vi "2.vi"() -> ()   [LabVIEW 2018]
uses:
  <vilib>/DAQmx/read.llb/DAQmx Read (Analog DBL 1Chan 1Samp).vi
  <vilib>/DAQmx/write.llb/DAQmx Write (Digital Bool 1Line 1Point).vi
  <vilib>/DAQmx/create/channels.llb/DAQmx Create Channel (AI-Voltage-Basic).vi
  <vilib>/DAQmx/create/channels.llb/DAQmx Create Channel (DO-Digital Output).vi
  <vilib>/DAQmx/miscellaneous.llb/DAQmx Fill In Error Info.vi
panel:
  out "采集电压":dbl(graph)
  in  "下限":dbl format="%#_13g"
  in  "lines":tag
  in  "停止":bool
  out "提示":string
  out "报警灯":bool=TRUE
  in  "上限":dbl format="%#_13g"
  in  "physical channels":tag caption="物理通道"
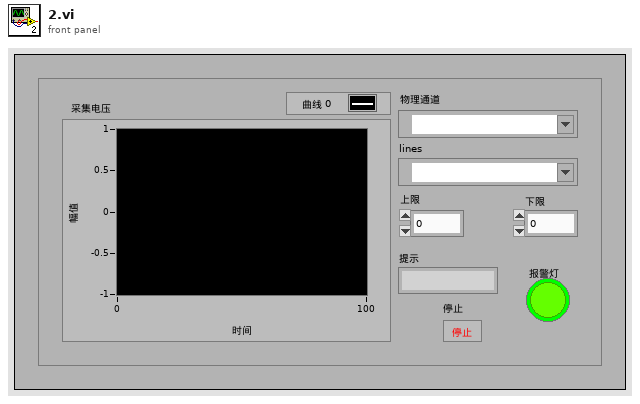
[diagram p1: front panel]
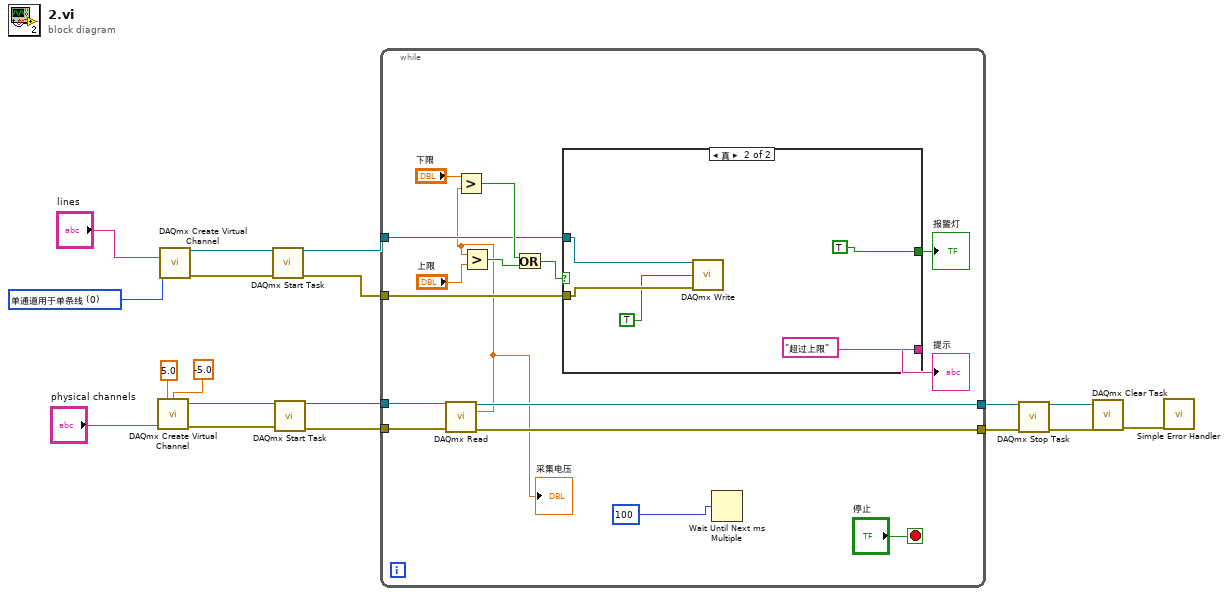
[diagram p0: block diagram]
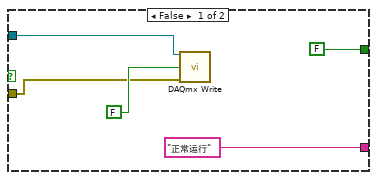
[diagram p2: hidden frame]
diagram:
  w3 = 0 items=["单通道用于单条线", "单通道用于所有线"] ("line grouping")
  n1 = call-poly <vilib>:"DAQmx Create Virtual Channel.vi"("maximum value"=5.0, "minimum value"=-5.0, "physical channels"="physical channels") -> ("task out"=w16:refnum<k21>, "error out"=w17:errorcluster)  [unwired: 11 in]
  n2 = call-poly <vilib>:"DAQmx Create Virtual Channel.vi"("lines"="lines", "line grouping"=w3) -> ("task out"=w6:refnum<k21>, "error out"=w5:errorcluster)  [unwired: 12 in]
  n3 = call <vilib>:"DAQmx Start Task.vi"("task/channels in"=w6, "error in"=w5) -> ("task out"=w1:refnum<k21>, "error out"=w2:errorcluster)  [unwired: 12 in]
  n4 = call <vilib>:"DAQmx Start Task.vi"("task/channels in"=w16, "error in"=w17) -> ("task out"=w14:refnum<k21>, "error out"=w15:errorcluster)  [unwired: 12 in]
  n5 = while {
    tunnel: w15 -> [w34]
    tunnel: w14 -> [w33]
    tunnel: [w30] -> w13
    tunnel: [w32] -> w11
    tunnel: w2 -> [w28]
    tunnel: w1 -> [w22]
    stop <- "停止" stop-if-true
    n6 = call-poly <vilib>:"DAQmx Read.vi"("task/channels in"=w33, "error in"=w34) -> ("task out"=w30:refnum<k21>, "data"=w20:dbl, "error out"=w32:errorcluster)  [unwired: 11 in]
    "采集电压" <- w20
    n7 = Greater?(x="下限", y=w20) -> (0:w25:bool)
    n8 = Greater?(x=w20, y="上限") -> (0:w24:bool)
    n9 = Or(x=w25, y=w24) -> (x .or. y?=w23:bool)
    n10 = case shown="真" w23 {
      tunnel: ["正常运行" "超过上限"] -> w29
      tunnel: w28 -> [w36 w43]
      tunnel: w22 -> [w37 w41]
      tunnel: [FALSE TRUE] -> w19
      frame False {
        n11 = call-poly <vilib>:"DAQmx Write.vi"("task/channels in"=w37, "data"=FALSE, "error in"=w36) -> ()  [unwired: 10 in, 3 out]
      }
      frame True {
        n12 = call-poly <vilib>:"DAQmx Write.vi"("task/channels in"=w41, "data"=TRUE, "error in"=w43) -> ()  [unwired: 10 in, 3 out]
      }
    }
    "报警灯" <- w19
    "提示" <- w29
    n13 = Wait Until Next ms Multiple(millisecond multiple=100) -> ()  [unwired: 1 out]
  }
  n14 = call <vilib>:"DAQmx Stop Task.vi"("task/channels in"=w13, "error in"=w11) -> ("task out"=w12:refnum<k21>, "error out"=w10:errorcluster)  [unwired: 12 in]
  n15 = call <vilib>:"DAQmx Clear Task.vi"("task in"=w12, "error in"=w10) -> ("error out"=w9:errorcluster)  [unwired: 13 in]
  n16 = call <vilib>:"Simple Error Handler.vi"("error in (no error)"=w9) -> ()  [unwired: 4 in, 5 out]
